vi "valves_opmode.vi"(0 "COM4 in":refnum<k24>, 5 "error in":errorcluster) -> (6 "COM4 out":refnum<k24>, 8 "error out":errorcluster)   [LabVIEW 2018]
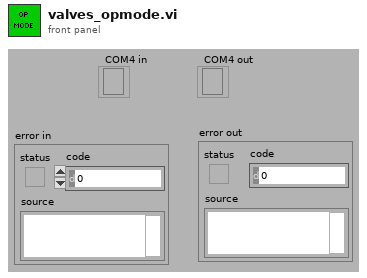
[diagram p1: front panel]
types:
  T1 = cluster{"Op A":u8[], "Op B":u8[], "Op C":u8[], "open":u8[], "L 3 A":u8[], "L 4 A 16":u8[], "F1 A":u8[], "L 4 A 34":u8[], "L 4 A 5":u8[], "FPw1 A":u8[], "L 2 A":u8[], "L 1 C FS":u8[], "L 2 C FS":u8[], "L 4 C 456 FS":u8[], "L 4 C 123 FS":u8[], "L 1 A":u8[], "L 1 C":u8[], "L 2 C":u8[], "L 4 C 456":u8[], "L 4 C 123":u8[], "FPw1 C":u8[], "F1 B":u8[], "F1 C":u8[], "F2 C":u8[], "F5 C":u8[]}
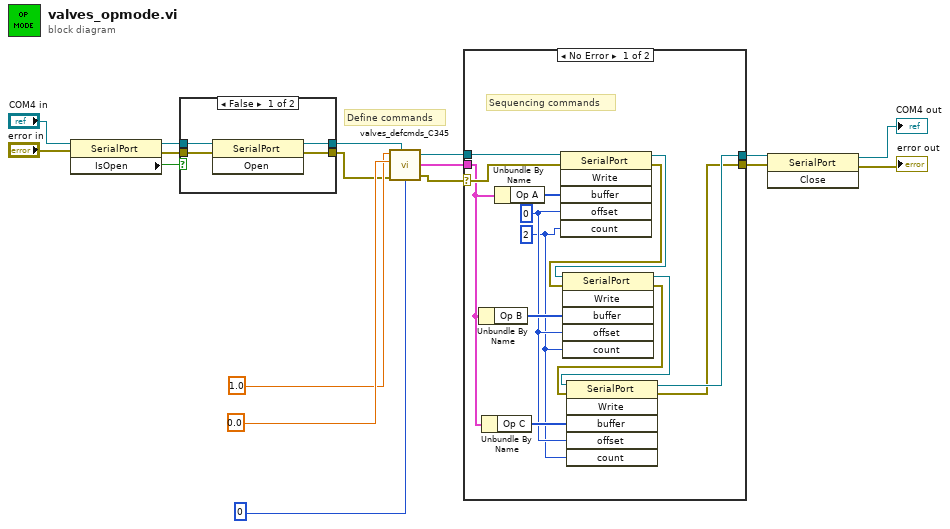
[diagram p0: block diagram]
diagram:
  # "Define commands"
  n1 = property class="SerialPort"(reference="COM4 in", error in="error in") -> (reference out=w9:refnum<k24>, error out=w10:errorcluster, "IsOpen"=w11:bool)
  n2 = case shown="False" w11 {
    tunnel: [w18 w23] -> w6
    tunnel: [w19 w22] -> w5
    tunnel: w10 -> [w20 w22]
    tunnel: w9 -> [w21 w23]
    frame False {
      n3 = invoke class="SerialPort" method="Open"(reference=w21, error in=w20) -> (reference out=w18:refnum<k24>, error out=w19:errorcluster)  [unwired: 1 in, 1 out]
    }
    frame True {
    }
  }
  n4 = call "valves_defcmds_C345.vi"("Input solution"=1.0, "Add to C"=0.0, "Rings to open"=u32 0, "error in"=w5, "COM4 in"=w6) -> ("COM4 out"=w15:refnum<k24>, "Commands out"=w16:T1, "error out"=w17:errorcluster)
  n5 = case shown="No Error" w17 {
    selector: w17 -> [w32 w39]
    tunnel: w15 -> [w37 w38]
    tunnel: [w29 w39] -> w3
    tunnel: w16 -> [w31 _]
    tunnel: [w30 w38] -> w4
    frame No Error {
      w24 = 2 ("count")
      w25 = 0 ("offset")
      # "Sequencing commands"
      n6 = Unbundle By Name(w31) -> ("Op B"=w27:u8[])
      n7 = Unbundle By Name(w31) -> ("Op C"=w28:u8[])
      n8 = Unbundle By Name(w31) -> ("Op A"=w26:u8[])
      n9 = invoke class="SerialPort" method="Write"(reference=w37, error in=w32, "buffer"=w26, "offset"=w25, "count"=w24) -> (reference out=w36:refnum<k24>, error out=w35:errorcluster)  [unwired: 1 in, 4 out]
      n10 = invoke class="SerialPort" method="Write"(reference=w36, error in=w35, "buffer"=w27, "offset"=w25, "count"=w24) -> (reference out=w34:refnum<k24>, error out=w33:errorcluster)  [unwired: 1 in, 4 out]
      n11 = invoke class="SerialPort" method="Write"(reference=w34, error in=w33, "buffer"=w28, "offset"=w25, "count"=w24) -> (reference out=w30:refnum<k24>, error out=w29:errorcluster)  [unwired: 1 in, 4 out]
    }
    frame Error {
    }
  }
  n12 = invoke class="SerialPort" method="Close"(reference=w4, error in=w3) -> (reference out=→"COM4 out":refnum<k24>, error out=→"error out":errorcluster)  [unwired: 1 in, 1 out]
